vi "PinMapService GetPinMap.vi"(6 "contextId":T1, 8 "error in":errorcluster, 9 "timeout (ms)":i32=-1, 10 "Request Data":T3, 11 "gRPC ID":T1) -> (0 "error out":errorcluster, 2 "Response Data":T2, 3 "gRPC ID out":T1)   [LabVIEW 2020, in "Pin Map_client.lvlib"]
uses:
  Pin Map_client.lvlib
  <vilib>/gRPC/LabVIEW gRPC Library/Shared/grpcId.ctl
  RPC Messages/ni_measurementlink_pinmap_v1_GetPinMapRequest.ctl
  RPC Messages/ni_measurementlink_pinmap_v1_PinMap.ctl
  14035477-4c25-4107-8ed5-d0c4ef420ce5.vi
  <vilib>/gRPC/LabVIEW gRPC Library/Shared/TranslateGrpcError.vi
  <vilib>/gRPC/LabVIEW gRPC Library/Shared/Wait On Occurence.vi
  <vilib>/gRPC/LabVIEW gRPC Library/Server API/Server/Get Server DLL Path.vi
  <vilib>/Utility/error.llb/Error Cluster From Error Code.vi
  <vilib>/gRPC/LabVIEW gRPC Library/grpc-lvsupport-release.lvlib
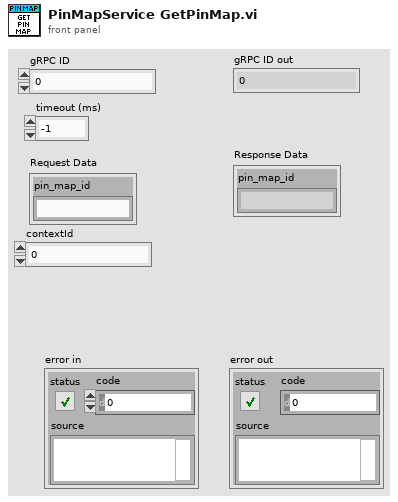
[diagram p1: front panel]
types:
  T1 = typedef "grpc-lvsupport-release.lvlib/grpcId.ctl" = u64
  T2 = typedef "Pin Map_client.lvlib/ni_measurementlink_pinmap_v1_PinMap.ctl" = cluster{"pin_map_id":string}
  T3 = typedef "Pin Map_client.lvlib/ni_measurementlink_pinmap_v1_GetPinMapRequest.ctl" = cluster{"pin_map_id":string}
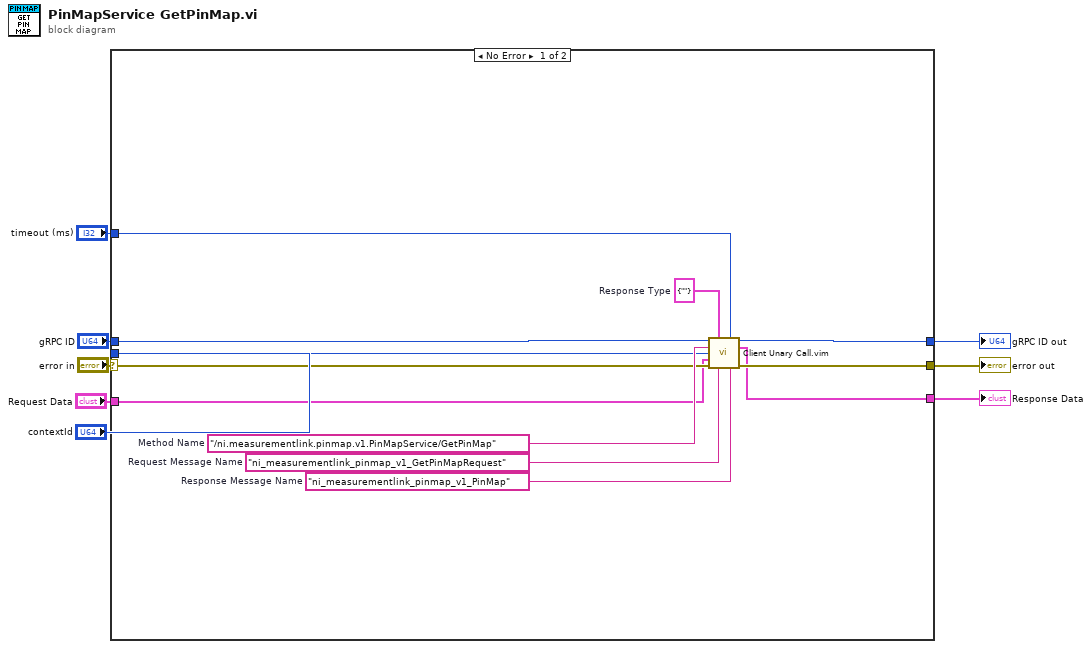
[diagram p0: block diagram]
diagram:
  n1 = case shown="No Error" "error in" {
    selector: "error in" -> [w16 w21]
    tunnel: [w15 w21] -> w7
    tunnel: "gRPC ID" -> [w14 w22]
    tunnel: [w13 w22] -> w5
    tunnel: "Request Data" -> [w12 _]
    tunnel: [w11 _] -> w3
    tunnel: "timeout (ms)" -> [w10 _]
    tunnel: "contextId" -> [w9 _]
    frame No Error {
      w17 = "ni_measurementlink_pinmap_v1_PinMap"  # Response Message Name
      w18 = "ni_measurementlink_pinmap_v1_GetPinMapRequest"  # Request Message Name
      w19 = T2 {"pin_map_id"=""}  # Response Type
      w20 = "/ni.measurementlink.pinmap.v1.PinMapService/GetPinMap"  # Method Name
      n2 = call "Client Unary Call.vim"("ClientID in"=w14, "Response Type"=w19, "timeout (ms)"=w10, "Method Name"=w20, "contextId"=w9, "Request Data"=w12, "error in"=w16, "Request Message Name"=w18, "Response Message Name"=w17) -> ("ClientID out"=w13:u64, "Response Data"=w11:T2, "error out"=w15:errorcluster)  [unwired: 4 in]
    }
    frame Error {
    }
  }
  "error out" <- w7
  "gRPC ID out" <- w5
  "Response Data" <- w3
